vi "RingControlDemo.vi"() -> ()   [LabVIEW 2018]
panel:
  out "Ring Idex":dbl
  out "Ring Value":string
  in  "Class Selection - Menu Ring":u16(ring) items=["Physics", "Math", "Language Arts", "History"]
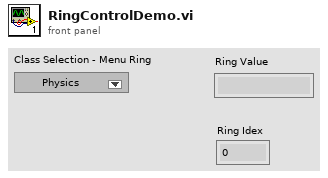
[diagram p1: front panel]
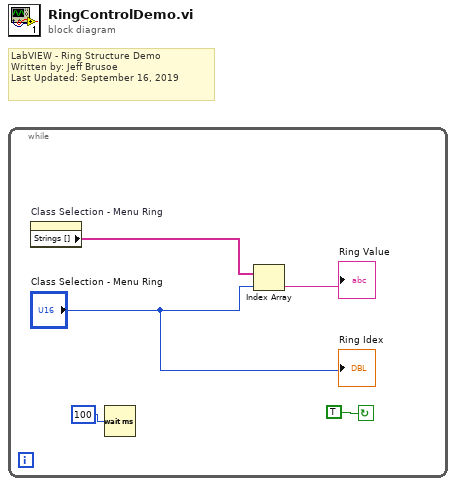
[diagram p0: block diagram]
diagram:
  # "LabVIEW - Ring Structure Demo\nWritten by: Jeff Brusoe\nLast Updated: September 16, 2019"
  n1 = while {
    stop <- TRUE continue-if-true
    n2 = property on="Class Selection - Menu Ring" class="Ring (strict)"() -> ("Strings []"=w4:string[])  [unwired: 2 in, 2 out]
    n3 = Wait (ms)(milliseconds to wait=u32 100) -> ()  [unwired: 1 out]
    n4 = Index Array(array=w4, index="Class Selection - Menu Ring") -> (element=→"Ring Value":string)
    "Ring Idex" <- "Class Selection - Menu Ring"
  }
